vi "GetU16ImageArray.vi"(8 "error in (no error)":errorcluster) -> (0 "error out":errorcluster, 2 "OutputPixels":u16[](array[numeric]), 3 "Image Pixels":u16[][](array[numeric]), 4 "return":i32)   [LabVIEW 2015]
uses:
  [Global] Image.vi
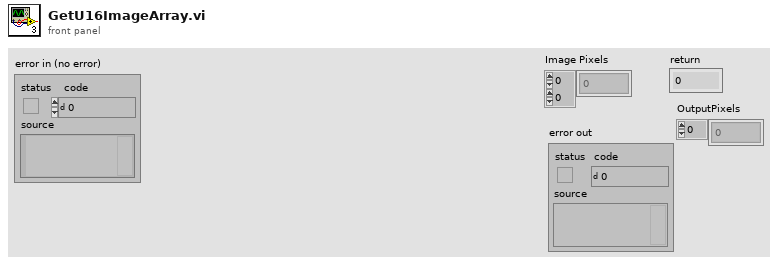
[diagram p1: front panel]
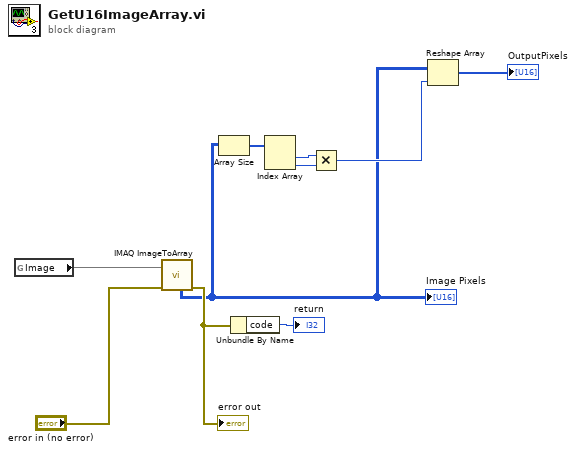
[diagram p0: block diagram]
diagram:
  n1 = global read "[Global] Image.vi" "Image"() -> (w10)
  n2 = call "IMAQ ImageToArray"("error in (no error)"="error in (no error)", "Image"=w10) -> ("Image Pixels (U16)"=w2:u16[][], "error out"=w8:errorcluster)  [unwired: 2 in, 3 out]
  "Image Pixels" <- w2
  "error out" <- w8
  n3 = Array Size(array=w2) -> (size(s)=w6:i32[])
  n4 = Unbundle By Name(w8) -> ("code"=→"return":i32)
  n5 = Index Array(array=w6) -> (element #1=w4:i32, element #2=w5:i32)  [unwired: 2 in]
  n6 = Multiply(x=w4, y=w5) -> (x*y=w3:i32)
  n7 = Reshape Array(w2, w3) -> (→"OutputPixels":u16[])
